vi "Set Event Timing Windows.vi"(8 "error in (no error)":errorcluster, 10 "Windows":T2[](array[typedef]), 11 "Item Ref in":T1 format="%.0x") -> (0 "error out":errorcluster, 3 "Item Ref out":T1 format="%.0x")   [LabVIEW 2017, in "Engine Simulation Toolkit System Explorer.lvlib"]
uses:
  Engine Simulation Toolkit System Explorer.lvlib
  Event Timing Window.ctl
  <vilib>/NI Veristand/Custom Device API/Custom Device Item Ref.ctl
  Shared/Properties.vi
  <vilib>/NI Veristand/Custom Device API/Set Item Property (Double Array).vi
  <vilib>/NI Veristand/Custom Device API/Set Item Property (String Array).vi
  Shared/Engine Simulation Toolkit Shared.lvlib
  <vilib>/NI Veristand/Custom Device API/Custom Device API.lvlib
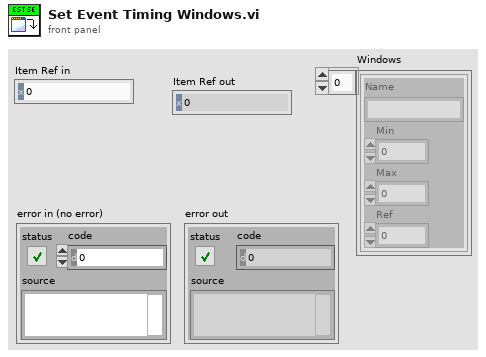
[diagram p1: front panel]
types:
  T1 = typedef "Custom Device API.lvlib/Custom Device Item Ref.ctl" = u64
  T2 = typedef "Engine Simulation Toolkit System Explorer.lvlib/Event Timing Window.ctl" = cluster{"Name":string, "Min":dbl, "Max":dbl, "Ref":dbl}
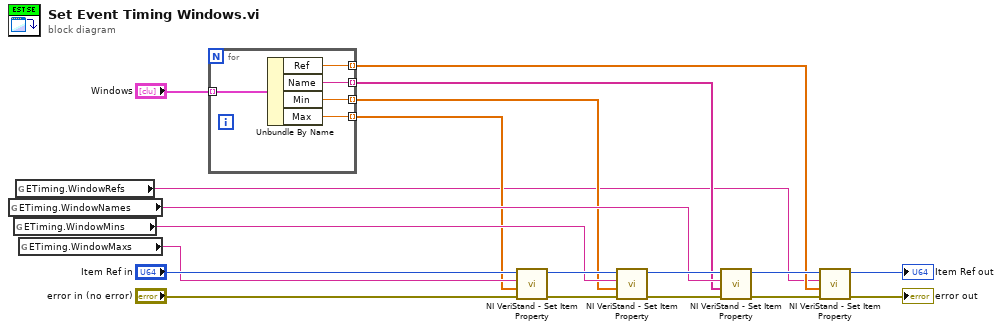
[diagram p0: block diagram]
diagram:
  n1 = global read "Properties.vi" "ETiming.WindowNames"() -> (w11:string)
  n2 = global read "Properties.vi" "ETiming.WindowMins"() -> (w14:string)
  n3 = global read "Properties.vi" "ETiming.WindowRefs"() -> (w1:string)
  n4 = global read "Properties.vi" "ETiming.WindowMaxs"() -> (w17:string)
  n5 = for {
    tunnel: "Windows" -> [w24] mode=indexing
    tunnel: [w23] -> w9 mode=indexing
    tunnel: [w22] -> w8 mode=indexing
    tunnel: [w21] -> w7 mode=indexing
    tunnel: [w20] -> w2 mode=indexing
    n6 = Unbundle By Name(w24) -> ("Ref"=w20:dbl, "Name"=w21:string, "Min"=w22:dbl, "Max"=w23:dbl)
  }
  n7 = call-poly <vilib>:"NI VeriStand - Set Item Property.vi"("error in (no error)"="error in (no error)", "Value"=w9, "Property Name"=w17, "Item Ref in"="Item Ref in") -> ("error out"=w15:errorcluster, "Item Ref out"=w16:T1)  [unwired: 5 in, 1 out]
  n8 = call-poly <vilib>:"NI VeriStand - Set Item Property.vi"("error in (no error)"=w15, "Value"=w8, "Property Name"=w14, "Item Ref in"=w16) -> ("error out"=w12:errorcluster, "Item Ref out"=w13:T1)  [unwired: 5 in, 1 out]
  n9 = call-poly <vilib>:"NI VeriStand - Set Item Property.vi"("error in (no error)"=w12, "Value"=w7, "Property Name"=w11, "Item Ref in"=w13) -> ("error out"=w5:errorcluster, "Item Ref out"=w6:T1)  [unwired: 5 in, 1 out]
  n10 = call-poly <vilib>:"NI VeriStand - Set Item Property.vi"("error in (no error)"=w5, "Value"=w2, "Property Name"=w1, "Item Ref in"=w6) -> ("error out"=→"error out":errorcluster, "Item Ref out"=→"Item Ref out":T1)  [unwired: 5 in, 1 out]
